vi "zipSingleFile.vi"(9 "zip folderFile":path, 11 "source file path":path) -> (0 "error out":errorcluster)   [LabVIEW 2012]
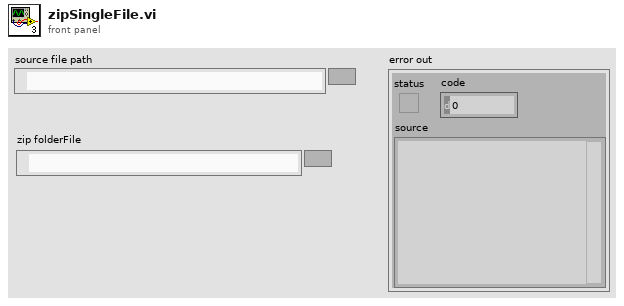
[diagram p1: front panel]
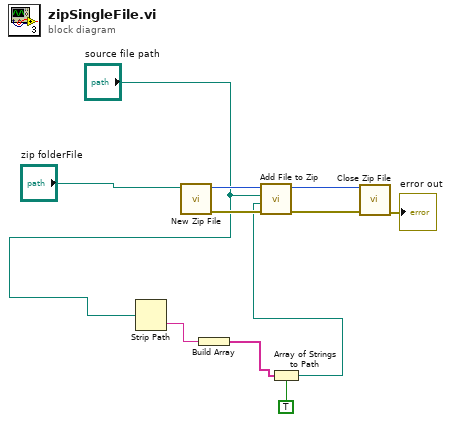
[diagram p0: block diagram]
diagram:
  n1 = Strip Path(path="source file path") -> (name=w3:string)  [unwired: 1 out]
  n2 = call <vilib>:"New Zip File.vi"("target"="zip folderFile") -> ("error out"=w7:errorcluster, "zip file out"=w11:i64)  [unwired: 4 in, 1 out]
  n3 = Build Array(w3) -> (w2:string[])
  n4 = Array of Strings to Path(0:w2, 1:TRUE ("relative")) -> (2:w5:path)
  n5 = call <vilib>:"Add File to Zip.vi"("error in (no error)"=w7, "destination path in zip"=w5, "source file path"="source file path", "zip file in"=w11) -> ("error out"=w10:errorcluster, "zip file out"=w9:i64)  [unwired: 6 in]
  n6 = call <vilib>:"Close Zip File.vi"("error in (no error)"=w10, "zip file in"=w9) -> ("error out"=→"error out":errorcluster)  [unwired: 5 in]
